vi "Enter set motor speed in rpm.vi"(8 "error in (no error)":errorcluster, 10 "Motor speed (10rpm)":u16=10, 11 "VISA resource name":refnum<visa-resource-name>) -> (0 "error out":errorcluster, 3 "VISA resource name out":refnum<visa-resource-name>)   [LabVIEW 2018]
panel:
  out "resulting string":string
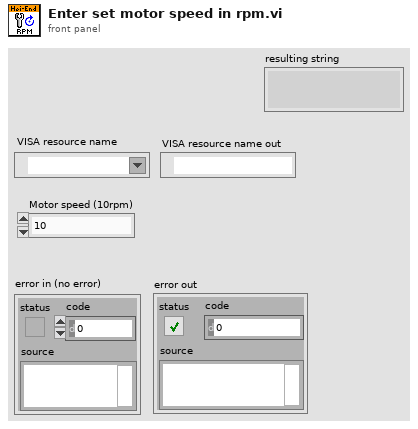
[diagram p1: front panel]
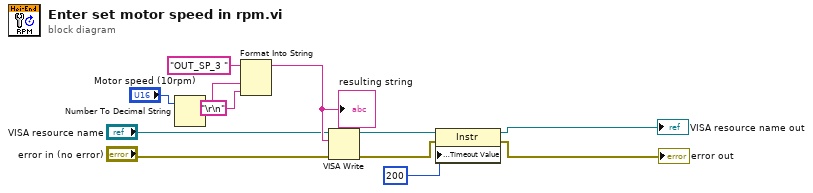
[diagram p0: block diagram]
diagram:
  n1 = Number To Decimal String(number="Motor speed (10rpm)") -> (decimal integer string=w1:string)  [unwired: 1 in]
  n2 = Format Into String(initial string="OUT_SP_3 ", w1, "\r\n") -> (resulting string=w11:string)  [unwired: 2 in, 1 out]
  "resulting string" <- w11
  n3 = VISA Write(VISA resource name="VISA resource name", write buffer=w11, error in (no error)="error in (no error)") -> (VISA resource name out=w6:refnum<visa-resource-name>, error out=w4:errorcluster)  [unwired: 1 out]
  n4 = property class="Instr"(reference=w6, error in=w4, "General Settings:Timeout Value"=u32 200) -> (reference out=→"VISA resource name out":refnum<visa-resource-name>, error out=→"error out":errorcluster)
